vi "Get Win Handle.vi"(8 "error in (no error)":errorcluster, 11 ".NET Refnum in":refnum<k24>) -> (0 "error out":errorcluster, 1 "Cluster":cluster{"Width":i32, "Height":i32}, 2 "Bounds":T1, 3 "ToInt32":i32)   [LabVIEW 2025, in "Test Unit.lvlib"]
uses:
  Test Unit.lvlib
  System.Windows.Forms
  System.Drawing
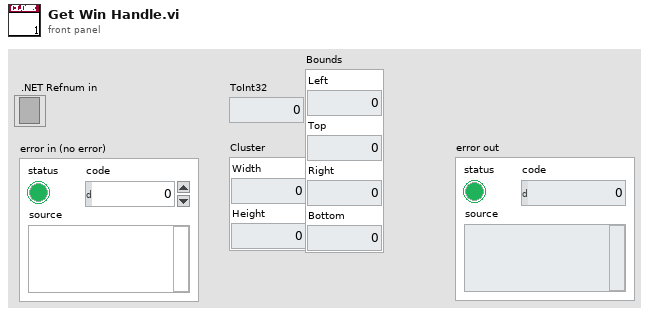
[diagram p1: front panel]
types:
  T1 = cluster{"Left":i32, "Top":i32, "Right":i32, "Bottom":i32}
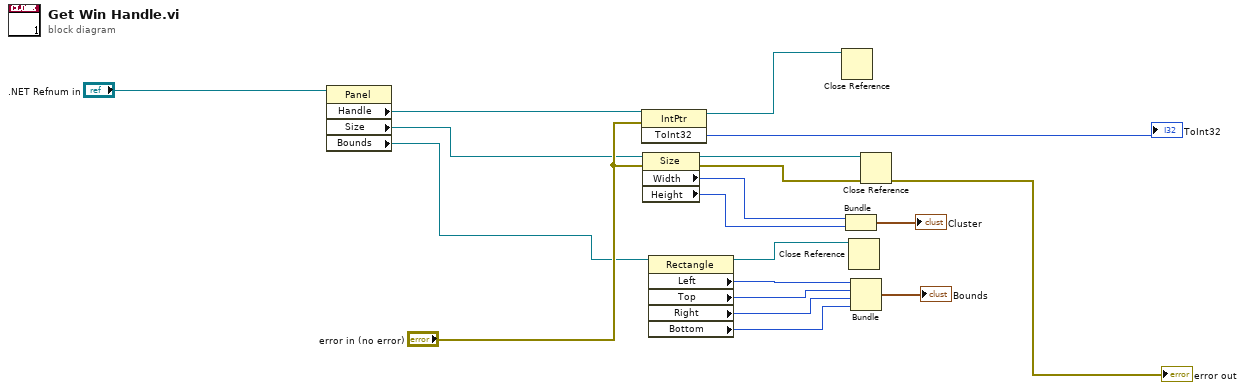
[diagram p0: block diagram]
diagram:
  n1 = property class="Panel"(reference=".NET Refnum in") -> ("Handle"=w11:refnum<k24>, "Size"=w14:refnum<k24>, "Bounds"=w9:refnum<k24>)  [unwired: 1 in, 2 out]
  n2 = invoke class="IntPtr" method="ToInt32"(reference=w11, error in="error in (no error)") -> (reference out=w12:refnum<k24>, "ToInt32"=→"ToInt32":i32)  [unwired: 1 in, 1 out]
  n3 = property class="Size"(reference=w14, error in="error in (no error)") -> (reference out=w15:refnum<k24>, error out=w2:errorcluster, "Width"=w16:i32, "Height"=w17:i32)
  n4 = property class="Rectangle"(reference=w9) -> (reference out=w4:refnum<k24>, "Left"=w8:i32, "Top"=w7:i32, "Right"=w6:i32, "Bottom"=w5:i32)  [unwired: 1 in, 1 out]
  n5 = Close Reference(reference=w12) -> ()  [unwired: 1 in, 1 out]
  n6 = Bundle("Width"=w16, "Height"=w17) -> (→"Cluster":cluster{"Width":i32, "Height":i32})  [unwired: 1 in]
  n7 = Close Reference(reference=w4) -> ()  [unwired: 1 in, 1 out]
  n8 = Bundle("Left"=w8, "Top"=w7, "Right"=w6, "Bottom"=w5) -> (→"Bounds":T1)  [unwired: 1 in]
  n9 = Close Reference(reference=w15, error in (no error)=w2) -> (error out=→"error out":errorcluster)
